vi "Telecommunications Parametric Testing.vi"() -> ()   [LabVIEW 2012]
doc: "The T1 Parametric testing application performs parametric testing of T1 signals. The T1 signal is a 1.544 Mb/s pulsed digital signal formed by multiplexing 24 voice channels. Each channel is sampled at 8000 samples/sec. Each sample is then converted to 8 bits using Pulse Coded Multiplexing. The 24 channels are then time-division multiplexed. Each frame, which corresponds to one sampling period, contains 192 bits ( 8 times 24) plus one bit for frame synchronization. Since frames occur at 8000 times per second, the bit rate is 1.544 Mb/s\n\nThis application performs the following parametric tests on T1 signals:\n\n1. Mask Test: Compares T1 signals with standard masks. The type of masks that are supported are ITU G.703 mask, EIA/TIA 547 and ANSI T1.102. The graph shows the mask in grey, the actual signal in green and failures as red squares. A boolean indicates whether the signal passed or failed the mask test and the indicator Number of Hits shows the number of times the signal did not pass the mask test.\n\n2. Measure T1 signal amplitude : Measures the amplitude of the T1 signal. The peak amplitude is displayed in the indicator Measured Amplitude.\n\n3. Measure T1 signal frequency : Measures the frequency of the T1 signal. The signal frequency in MHz is displayed in the indicator Measured Frequency.\n\nIn order for the Telecommunications Parametric Testing demo to work properly, Telecommunications Parametric Testing.llb, Telecommunications Parametric Testing.mdb, and Telecommunications Parametric Testing.udl must be in the same directory."
uses:
  Connection.llb/DB Tools Open Connec (Path).vi
  NI_Database_API_64.lvlib
panel:
  in  "Quit":bool
  in  "Launch Retrieve\nfrom Database VI":bool
  in  "Launch Test/Log\nto Database VI":bool
  # "Telecommunications Parametric Testing"
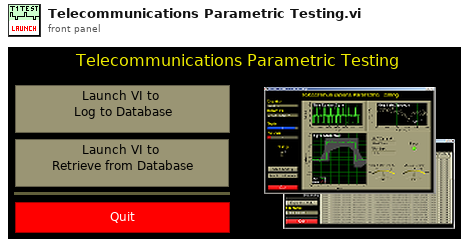
[diagram p1: front panel]
types:
  T1 = typedef "NI_Database_API_64.lvlib/Conn ObjectReference.ctl" = refnum<k1>
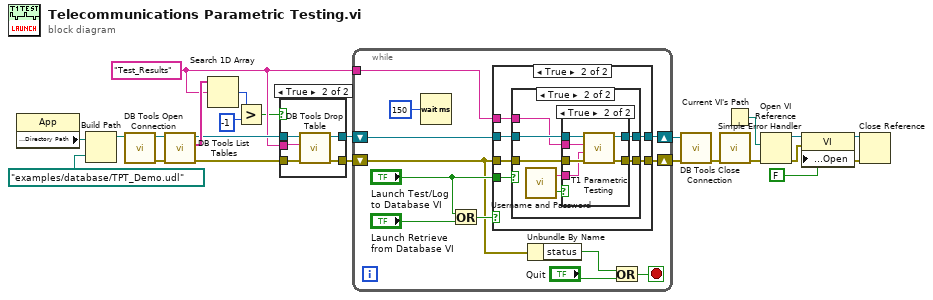
[diagram p0: block diagram]
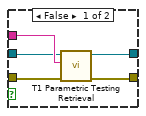
[diagram p3: hidden frame]
diagram:
  w8 = "Test_Results" ("element")
  n1 = property class="App"() -> ("Application:Directory Path"=w16:path)  [unwired: 2 in, 2 out]
  n2 = Build Path(base path=w16, name or relative path=path "examples/database/TPT_Demo.udl" ("Application:Directory Path")) -> (appended path=w14:path)
  n3 = call-poly "DB Tools Open Connection.vi"("connection information"=w14) -> ("error out"=w18:errorcluster, "connection reference"=w17:T1)  [unwired: 7 in]
  n4 = call "DB Tools List Tables.vi"("error in (no error)"=w18, "connection reference"=w17) -> ("error out"=w12:errorcluster, "tables"=w19:string[], "connection reference out"=w11:T1)  [unwired: 3 in]
  n5 = Search 1D Array(1D array=w19, element=w8) -> (index of element=w10:i32)  [unwired: 1 in]
  n6 = Greater?(x=w10, y=-1) -> (0:w1:bool)
  n7 = case shown="True" w1 {
    tunnel: w11 -> [w26 w30]
    tunnel: w12 -> [w25 w31]
    tunnel: [w26 w29] -> w6
    tunnel: [w25 w28] -> w7
    tunnel: w8 -> [_ w27]
    frame False {
    }
    frame True {
      n8 = call "DB Tools Drop Table.vi"("error in (no error)"=w31, "table"=w27, "connection reference"=w30) -> ("error out"=w28:errorcluster, "connection reference out"=w29:T1)  [unwired: 5 in]
    }
  }
  n9 = while {
    shift-left: w7 -> [w34]
    shift-right: [w36] -> w4
    shift-left: w6 -> [w38]
    shift-right: [w37] -> w5
    tunnel: w8 -> [w39]
    stop <- w35 stop-if-true
    n10 = Wait (ms)(milliseconds to wait=u32 150) -> ()  [unwired: 1 out]
    n11 = Or(x="Launch Test/Log\nto Database VI", y="Launch Retrieve\nfrom Database VI") -> (x .or. y?=w40:bool)
    n12 = case shown="True" w40 {
      tunnel: "Launch Test/Log\nto Database VI" -> [_ w51]
      tunnel: w38 -> [w45 w50]
      tunnel: w34 -> [w44 w49]
      tunnel: [w45 w48] -> w37
      tunnel: [w44 w47] -> w36
      tunnel: w39 -> [_ w46]
      frame False {
      }
      frame True {
        n13 = case shown="True" w51 {
          tunnel: w50 -> [w55 w61]
          tunnel: w49 -> [w52 w60]
          tunnel: [w54 w59] -> w48
          tunnel: [w53 w58] -> w47
          tunnel: w46 -> [w56 w57]
          frame False {
            n14 = call "T1 Parametric Testing Retrieval.vi"("error in (no error)"=w52, "table name"=w56, "connection reference"=w55) -> ("error out"=w53:errorcluster, "connection reference out"=w54:T1)  [unwired: 3 in]
          }
          frame True {
            n15 = call "Username and Password.vi"() -> ("User name: 2"=w63:string, "Logged In?"=w62:bool)  [unwired: 1 in]
            n16 = case shown="True" w62 {
              tunnel: w63 -> [_ w66]
              tunnel: w61 -> [w65 w71]
              tunnel: w60 -> [w64 w70]
              tunnel: [w65 w69] -> w59
              tunnel: [w64 w68] -> w58
              tunnel: w57 -> [_ w67]
              frame False {
              }
              frame True {
                n17 = call "T1 Parametric Testing.vi"("error in"=w70, "Operator"=w66, "table name"=w67, "connection reference"=w71) -> ("error out"=w68:errorcluster, "connection reference out"=w69:T1)  [unwired: 3 in]
              }
            }
          }
        }
      }
    }
    n18 = Unbundle By Name(w34) -> ("status"=w33:bool)
    n19 = Or(x=w33, y="Quit") -> (x .or. y?=w35:bool)
  }
  n20 = call "DB Tools Close Connection.vi"("error in (no error)"=w4, "connection reference"=w5) -> ("error out"=w9:errorcluster)  [unwired: 5 in]
  n21 = call <vilib>:"Simple Error Handler.vi"("error in (no error)"=w9) -> ("error out"=w3:errorcluster)  [unwired: 4 in, 4 out]
  n22 = Current VI's Path() -> (path=w2:path)
  n23 = Open VI Reference(vi path=w2, error in (no error)=w3) -> (vi reference=w24:refnum<vi>, error out=w23:errorcluster)  [unwired: 4 in]
  n24 = property class="VI"(reference=w24, error in=w23, "Front Panel Window:Open"=FALSE) -> (reference out=w20:refnum<vi>, error out=w21:errorcluster)
  n25 = Close Reference(reference=w20, error in (no error)=w21) -> ()  [unwired: 1 out]
